vi "IMAQ FPGA CXP Wait For New Frame.vi"(10 "DV":bool, 11 "Reset":bool) -> (3 "Enable":bool)   [LabVIEW 2020]
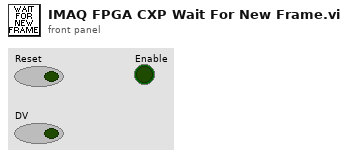
[diagram p1: front panel]
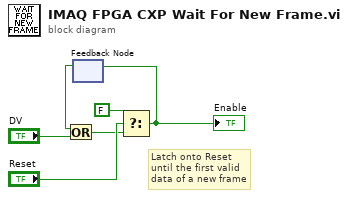
[diagram p0: block diagram]
diagram:
  # "Latch onto Reset\nuntil the first valid\ndata of a new frame"
  n1 = feedback #1() -> (w1:bool)  [unwired: 1 in]
  n2 = Or(x=w1, y="DV") -> (x .or. y?=w4:bool)
  n3 = Select(t=FALSE ("Reset"), s="Reset", f=w4) -> (s? t:f=w3:bool)
  "Enable" <- w3
  n4 = feedback-in #1(w3) -> ()
